vi "Configure Resume Trigger [RT].vi"(7 "Trigger Slope (Positive)":i32(ring) caption="trigger slope (Positive)" items=["Positive", "Negative", "Either"], 8 "error in (no error)":errorcluster, 9 "Trigger Source (None)":string(combo) caption="trigger source (None)", 10 "Channel Name (\"\")":string="CHANNEL1" caption="channel name (\"CHANNEL1\")", 11 "CS++Fgen in":refnum<class "CS++Fgen.lvclass">) -> (0 "error out":errorcluster, 3 "CS++Fgen out":refnum<class "CS++Fgen.lvclass">)   [LabVIEW 2016, in "CS++Fgen.lvlib" / "CS++Fgen.lvclass"]
doc: "This VI configures the properties that control the function generator's resume trigger. These properties are the resume trigger source and slope.\n\nA resume trigger resumes generation after it has been paused by a hold trigger, starting with the next point.\n\nNote:\n\n(1) This VI is part of the IviFgenResumeTrigger [RT] extension group."
uses:
  CS++Fgen.lvclass
  CSPP_Core/Classes/CS++ProcessVariables/ProcessVariable/PV.lvclass
  PV-Enum-n.ctl
  CSPP_Core/Classes/CS++ProcessVariables/ProcessVariable/PV.lvclass/PV.ctl
  CS++Fgen.lvclass/CS++Fgen.ctl
  CSPP_Core/Classes/CS++ProcessVariables/ProcessVariable/Write Data.vi
  CSPP_Core/Classes/CS++ProcessVariables/ProcessVariable/Write Timestamp.vi
  CSPP_Core/Classes/CS++ProcessVariables/ProcessVariable/Write Quality.vi
  CSPP_Core/Classes/CS++ProcessVariables/ProcessVariable/Write status.vi
  CSPP_Core/Classes/CS++ProcessVariables/PVConnection/PVConnection.lvclass
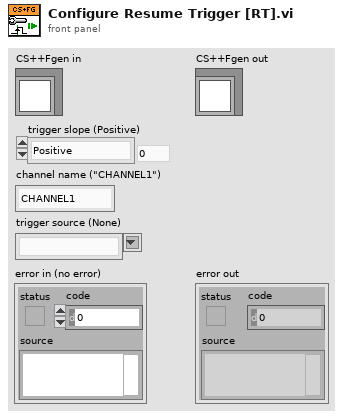
[diagram p1: front panel]
types:
  T1 = typedef "CS++Fgen.lvlib/CS++Fgen.lvclass/PV-Enum-n.ctl" = enum16{"Amplitude", "Arb-Frequency", "DCOffset", "Frequency", "OutputImpedance", "StartPhase", "AdvancedTriggerSlope", "AM-Source", "BurstCount", "FM-Source", "OperationMode", "ResumeTriggerSlope", "StartTriggerSlope", "StopTriggerSlope", "Waveform", "TriggerSource", "AM-Enabled", "ChannelEnabled", "FM-Enabled", "AdvancedTriggerSource", "ResumeTriggerSource", "StartTriggerSource", "StopTriggerSource"}
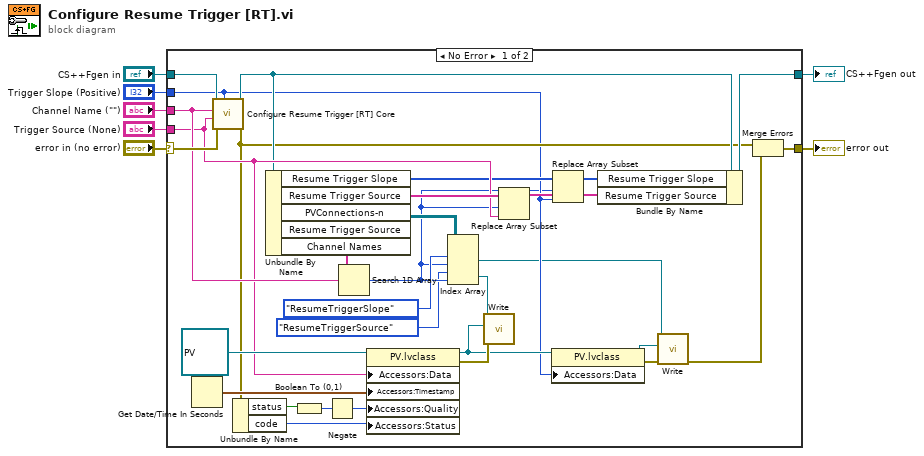
[diagram p0: block diagram]
diagram:
  n1 = case shown="No Error" "error in (no error)" {
    selector: "error in (no error)" -> [w37 w40]
    tunnel: [w21 w40] -> w6
    tunnel: [w23 w39] -> w4
    tunnel: "CS++Fgen in" -> [w38 w39]
    tunnel: "Trigger Slope (Positive)" -> [w15 _]
    tunnel: "Channel Name (\"\")" -> [w26 _]
    tunnel: "Trigger Source (None)" -> [w25 _]
    frame No Error {
      n2 = Get Date/Time In Seconds() -> (seconds since 1Jan1904=w36:timestamp)
      n3 = call-dynamic "Configure Resume Trigger [RT] Core.vi"("Trigger Slope (Positive)"=w15, "error in (no error)"=w37, "Trigger Source (None)"=w25, "Channel Name (\"\")"=w26, "CS++Fgen in"=w38) -> ("error out"=w22:errorcluster, "CS++Fgen out"=w24:refnum<class "CS++Fgen.lvclass">)  [unwired: 5 in]
      n4 = Unbundle By Name(w22) -> ("status"=w32:bool, "code"=w30:i32)
      n5 = Unbundle By Name(w24) -> ("Resume Trigger Slope"=w20:i32[], "Resume Trigger Source"=w28:string[], "PVConnections-n"=w14:refnum<class "PVConnection.lvclass">[][], "Channel Names"=w33:string[])  [unwired: 1 out]
      n6 = Boolean To (0,1)(Boolean=w32) -> (0, 1=w31:i16)
      n7 = Negate(x=w31) -> (-x=w29:i16)
      n8 = Search 1D Array(1D array=w33, element=w26) -> (index of element=w9:i32)  [unwired: 1 in]
      n9 = property class="PV.lvclass"(reference=refnum<class "PV.lvclass"> refnum ("PV"), "Accessors:Data"=w25, "Accessors:Timestamp"=w36, "Accessors:Quality"=w29, "Accessors:Status"=w30) -> (reference out=w16:refnum<class "PV.lvclass">, error out=w34:errorcluster)  [unwired: 1 in]
      n10 = Index Array(array=w14, index (row) #1=PV-Enum-n."ResumeTriggerSlope" ("PV-Enum-n"), index (col) #1=w9, index (row) #2=PV-Enum-n."ResumeTriggerSource" ("PV-Enum-n"), index (col) #2=w9) -> (element #1=w13:refnum<class "PVConnection.lvclass">, element #2=w10:refnum<class "PVConnection.lvclass">)
      n11 = call "Write.vi"("error in (no error)"=w34, "PV"=w16, "PVConnection in"=w10) -> ()  [unwired: 7 in, 2 out]
      n12 = Replace Array Subset(array=w28, new element=w25, index=w9) -> (w27:string[])
      n13 = property class="PV.lvclass"(reference=w16, "Accessors:Data"=w15) -> (reference out=w18:refnum<class "PV.lvclass">, error out=w17:errorcluster)  [unwired: 1 in]
      n14 = Replace Array Subset(array=w20, new element=w15, index=w9) -> (w19:i32[])
      n15 = Bundle By Name(cluster=w24, "Resume Trigger Slope"=w19, "Resume Trigger Source"=w27) -> (w23:refnum<class "CS++Fgen.lvclass">)
      n16 = call "Write.vi"("error in (no error)"=w17, "PV"=w18, "PVConnection in"=w13) -> ("error out"=w12:errorcluster)  [unwired: 7 in, 1 out]
      n17 = Merge Errors(w22, w12) -> (w21:errorcluster)
    }
    frame Error {
    }
  }
  "error out" <- w6
  "CS++Fgen out" <- w4
